vi "Function.vi"(8 "error in (no error)":errorcluster, 10 "Value":u8, 11 "Two Terminal in":refnum<class "Increment_U8.lvclass">) -> (0 "error out":errorcluster, 2 "Result":u8, 3 "Two Terminal out":refnum<class "Increment_U8.lvclass">)   [LabVIEW 2021, in "Increment_U8.lvclass"]
uses:
  Increment_U8.lvclass
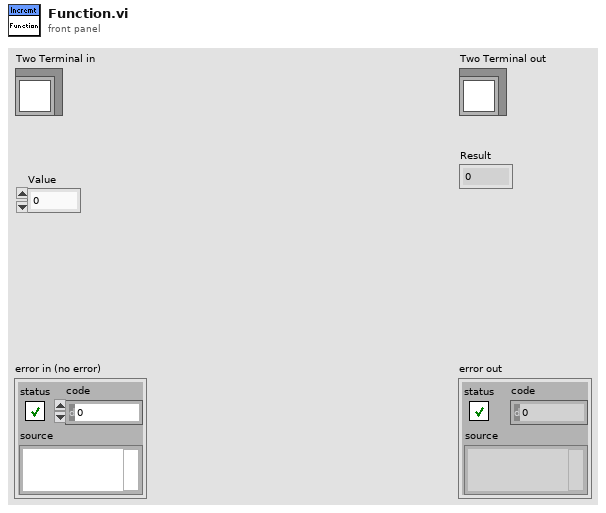
[diagram p1: front panel]
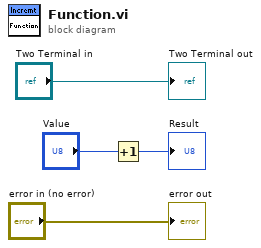
[diagram p0: block diagram]
diagram:
  n1 = Increment(x="Value") -> (x+1=→"Result":u8)
  "error out" <- "error in (no error)"
  "Two Terminal out" <- "Two Terminal in"
